vi "PS90_TargetMode.vi"(1 "Read?":bool, 5 "Value-In":i32 min=0 max=1, 6 "error in (no error)":errorcluster, 7 "Axis number":i32=1 min=1 max=9, 8 "Control unit ID":i32=1 min=1 max=10, 9 "DLOwis.lvclass":refnum<class "DLOwis.lvclass">) -> (0 "error out":errorcluster, 3 "DLOwis.lvclass":refnum<class "DLOwis.lvclass">, 4 "Value-Out":i32)   [LabVIEW 2018, in "DLOwis.lvclass"]
doc: "PS90_TargetMode.vi, created: 17.10.2006 alex; last change: 19.07.2016 alex;\n\n<B>FUNCTIONS:</B> \n\n<B>Read:</B> FALSE: read target mode of an axis.\n<B>Write:</B> TRUE: set target mode of an axis.\n----------------------------------------------------------------------------------------\n<B>INPUT:</B>\n[TF] <B>function:</B> function selector. (Read, Write)\n[I32] <B>Control unit ID:</B> control unit index. (Default=1, Range=1...10)\n[I32] <B>Axis number:</B> axis number. (Default=1, Range=1...9)\n[I32] <B>Value-In:</B> target mode. (only for Write: Default=0, Range=0...1)\n0 - relative positioning (target value is distance),\n1 - absolute positioning (target value is target position). \n[CLU] <B>error in</B>\n----------------------------------------------------------------------------------------\n<B>OUTPUT:</B>\n[I32] <B>Value-Out:</B> target mode. (for Write: Value-Out=Value-In)\n0 - relative positioning (target value is distance),\n1 - absolute positioning (target value is target position).\n[CLU] <B>error out</B>\n----------------------------------------------------------------------------------------\n<B>SUB-VIs:</B>\nPS90_GetReadError.vi\n----------------------------------------------------------------------------------------\n<B>EXT-Calls:</B>\nps90.dll (V2.00)\n----------------------------------------------------------------------------------------"
uses:
  DLOwis.lvclass
  C:/Dev/TRANCON/Classes/Delay Line/DelayLine.lvclass
  DelayLine.lvclass/DelayLine.ctl
  DelayLine.lvclass
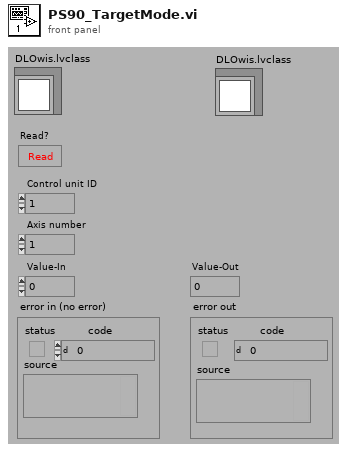
[diagram p1: front panel]
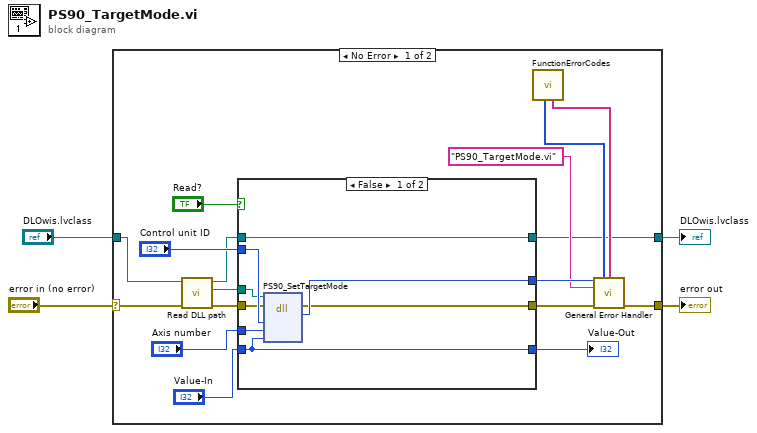
[diagram p0: block diagram]
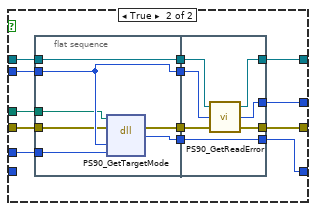
[diagram p2: hidden frame]
diagram:
  n1 = case shown="No Error" "error in (no error)" {
    selector: "error in (no error)" -> [w11 w57]
    tunnel: [w21 w57] -> w4
    tunnel: [w5 w58] -> w2
    tunnel: "DLOwis.lvclass" -> [w9 w58]
    frame No Error {
      n2 = call "Read DLL path.vi"("error in (no error)"=w11, "DelayLine in"=w9) -> ("error out"=w10:errorcluster, "DLL path"=w7:path, "DelayLine out"=w6:refnum<class "DLOwis.lvclass">)  [unwired: 7 in]
      n3 = case shown="False" "Read?" {
        tunnel: "Control unit ID" -> [w28 w41]
        tunnel: [w29 w42] -> w18
        tunnel: "Value-In" -> [w26 _]
        tunnel: [w26 w40] -> w16
        tunnel: "Axis number" -> [w27 w39]
        tunnel: w10 -> [w25 w38]
        tunnel: [w24 w37] -> w8
        tunnel: w7 -> [w23 w36]
        tunnel: w6 -> [w22 w35]
        tunnel: [w22 w30] -> w5
        frame False {
          n4 = dll-call lib="C:/Dev/TRANCON/DLL/ps90.dll" fn="PS90_SetTargetMode" label="PS90_Set\nTarget\nMode"(path in=w23, error in=w25, "Index"=w28, "AxisNr"=w27, "Value"=w26) -> (error out=w24:errorcluster, "Rückgabetyp"=w29:i32)  [unwired: 4 in, 1 out]
        }
        frame True {
          n5 = flat-sequence {
            tunnel: w41 -> [w49]
            tunnel: [w49] -> w34
            tunnel: [w48] -> w33
            tunnel: w39 -> [w47]
            tunnel: w38 -> [w46]
            tunnel: [w43] -> w32
            tunnel: w36 -> [w45]
            tunnel: w35 -> [w44]
            tunnel: [w44] -> w31
            tunnel: [w56] -> w42
            tunnel: w34 -> [w55]
            tunnel: [w52] -> w40
            tunnel: w33 -> [w52]
            tunnel: w32 -> [w53]
            tunnel: [w51] -> w37
            tunnel: w31 -> [w54]
            tunnel: [w50] -> w30
            frame #0 {
              n6 = dll-call lib="C:/Dev/TRANCON/DLL/ps90.dll" fn="PS90_GetTargetMode" label="PS90_Get\nTarget\nMode"(path in=w45, error in=w46, "Index"=w49, "AxisNr"=w47) -> (error out=w43:errorcluster, "Rückgabetyp"=w48:i32)  [unwired: 3 in, 1 out]
            }
            frame #1 {
              n7 = call "PS90_GetReadError.vi"("error in (no error)"=w53, "Control unit ID"=w55, "DLOwis.lvclass"=w54) -> ("error IO"=w51:errorcluster, "Read error"=w56:i32, "DLOwis.lvclass"=w50:refnum<class "DLOwis.lvclass">)
            }
          }
        }
      }
      "Value-Out" <- w16
      n8 = call "FunctionErrorCodes.vi"() -> ("[user-defined codes]"=w13:i32[], "[user-defined descriptions]"=w12:string[])  [unwired: 8 in]
      n9 = call <vilib>:"General Error Handler.vi"("[error code] (0)"=w18, "[user-defined codes]"=w13, "[user-defined descriptions]"=w12, "[error source] (\" \")"="PS90_TargetMode.vi" ("[error source] (\" \")"), "error in (no error)"=w8) -> ("error out"=w21:errorcluster)  [unwired: 6 in, 4 out]
    }
    frame Error {
    }
  }
  "error out" <- w4
  "DLOwis.lvclass" <- w2
